vi "Get Device Type.vi"(8 "Error In":errorcluster, 11 "Install LV Data":T1) -> (0 "Error Out":errorcluster, 2 "Device Type":string, 3 "Install LV Data":T1)   [LabVIEW 2020, in "LMH-LINX.lvlib"]
uses:
  LMH-LINX.lvlib
  Install LV Data.ctl
  Target Info.ctl
  NIC Info.ctl
  NIC Mode.ctl
  <vilib>/regexp/Match Regular Expression.xnode
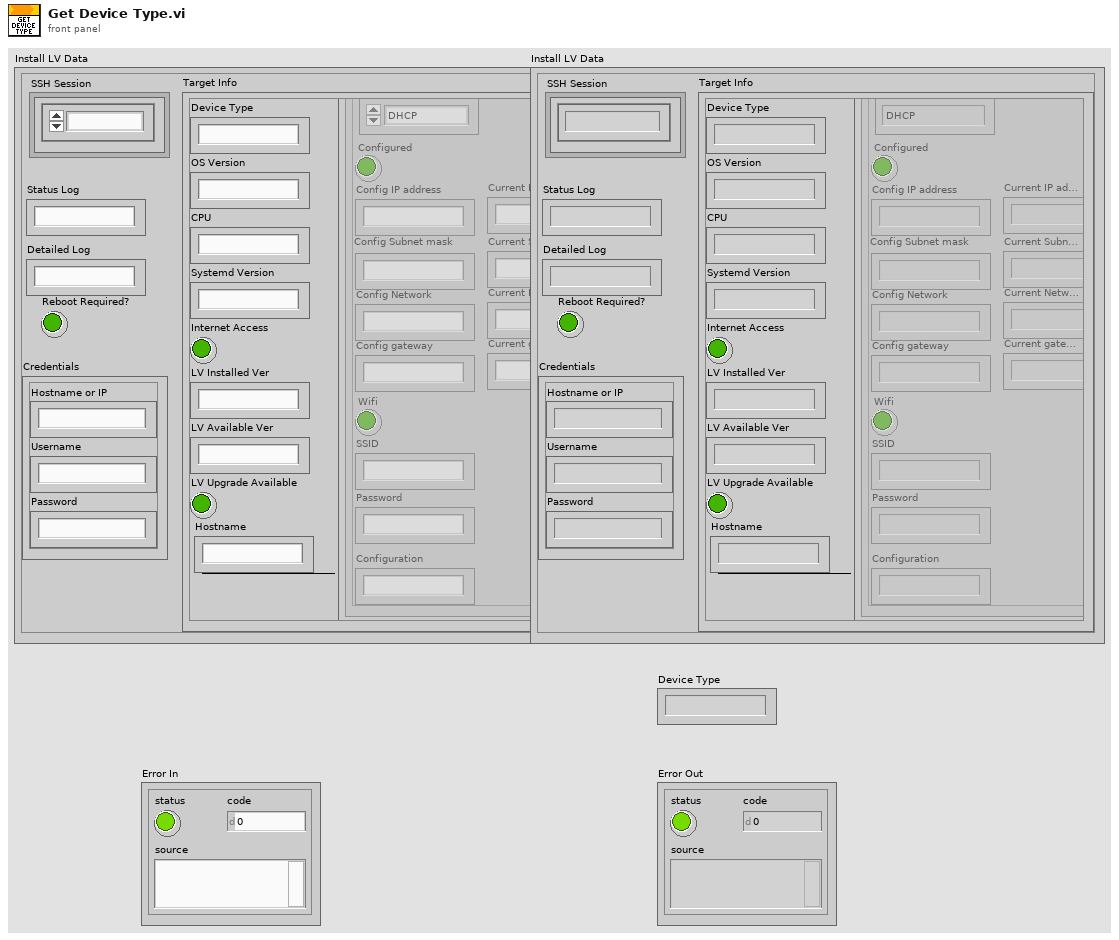
[diagram p1: front panel]
types:
  T1 = typedef "LMH-LINX.lvlib/Install LV Data.ctl" = cluster{"SSH Session":refnum<k1>, "Status Log":string, "Detailed Log":string, "Credentials":cluster{"Hostname or IP":string, "Username":string, "Password":string}, "Target Info":T2, "Reboot Required?":bool}
  T2 = typedef "LMH-LINX.lvlib/Target Info.ctl" = cluster{"OS Version":string, "CPU":string, "Systemd Version":string, "Internet Access":bool, "Device Type":string, "LV Installed Ver":string, "LV Available Ver":string, "LV Upgrade Available":bool, "Hostname":string, "NIC Info":T3[]}
  T3 = typedef "LMH-LINX.lvlib/NIC Info.ctl" = cluster{"Name":string, "NIC Mode":T4, "Configured":bool, "Config IP address":string, "Config Subnet mask":string, "Config Network":string, "Config gateway":string, "Wifi":bool, "SSID":string, "Password":string, "Configuration":string, "Current IP address":string, "Current Subnet mask":string, "Current gateway":string, "Current Network":string}
  T4 = typedef "LMH-LINX.lvlib/NIC Mode.ctl" = enum16{"DHCP", "Static", "Loopback"}
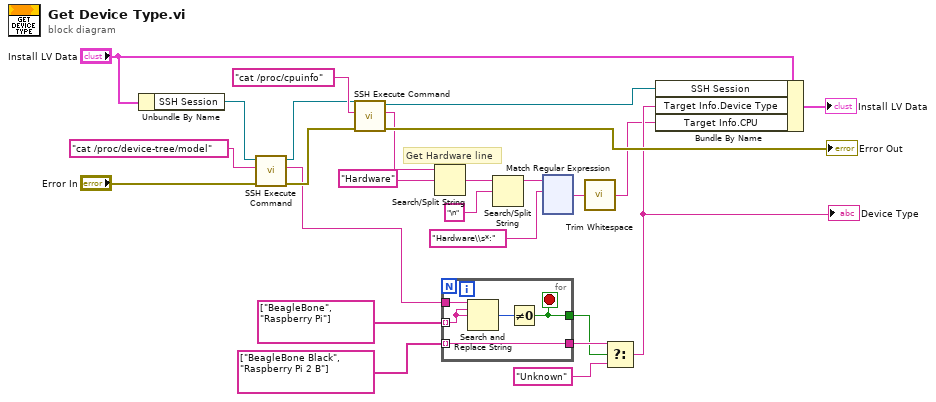
[diagram p0: block diagram]
diagram:
  # "Get Hardware line"
  n1 = Unbundle By Name("Install LV Data") -> ("SSH Session"=w4:refnum<k1>)
  n2 = call "SSH Execute Command.vi"("Error In"="Error In", "Command"="cat /proc/device-tree/model", "SSH Session"=w4) -> ("Error Out"=w3:errorcluster, "Std Out"=w1:string, "SSH Session"=w5:refnum<k1>)  [unwired: 6 in]
  n3 = call "SSH Execute Command.vi"("Error In"=w3, "Command"="cat /proc/cpuinfo", "SSH Session"=w5) -> ("Error Out"=→"Error Out":errorcluster, "Std Out"=w17:string, "SSH Session"=w23:refnum<k1>)  [unwired: 6 in]
  n4 = Search/Split String(string=w17, search string/char (-)="Hardware" ("regular expression")) -> (match + rest of string=w19:string)  [unwired: 1 in, 2 out]
  n5 = for {
    tunnel: w1 -> [w30]
    tunnel: string[] ["BeagleBone", "Raspberry Pi"] -> [w28] mode=indexing
    tunnel: [w26] -> w15
    tunnel: [w27] -> w14
    tunnel: string[] ["BeagleBone Black", "Raspberry Pi 2 B"] -> [w26] mode=indexing
    stop <- w27 stop-if-true
    n6 = Search and Replace String(input string=w30, search string=w28, replace string=w28) -> (number of replacements=w29:i32)  [unwired: 5 in, 3 out]
    n7 = Not Equal To 0?(x=w29) -> (x != 0?=w27:bool)
  }
  n8 = Search/Split String(string=w19, search string/char (-)="\n" ("regular expression")) -> (substring before match=w7:string)  [unwired: 1 in, 2 out]
  n9 = xnode "Match Regular Expression"("input string"=w7, "regular expression"="Hardware\\s*:") -> ("after match"=w8:string)  [unwired: 4 in, 4 out]
  n10 = call <vilib>:"Trim Whitespace.vi"("string"=w8) -> ("trimmed string"=w10:string)  [unwired: 1 in]
  n11 = Select(t=w15, s=w14, f="Unknown" ("regular expression")) -> (s? t:f=w11:string)
  "Device Type" <- w11
  n12 = Bundle By Name(cluster="Install LV Data", "SSH Session"=w23, "Target Info.Device Type"=w11, "Target Info.CPU"=w10) -> (→"Install LV Data":T1)
